vi "sub_angle-limit.vi"(11 "States Out":T1 format="%.4f") -> (3 "Off limit":bool)   [LabVIEW 2018]
uses:
  Model/States.ctl
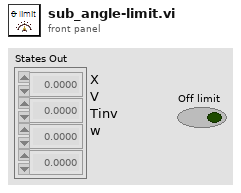
[diagram p1: front panel]
types:
  T1 = typedef "States.ctl" = dbl[]
  T2 = typedef "ctr-ref.ctl" = cluster{"connected":refnum<vi>, "start":refnum<vi>, "read_data":refnum<vi>, "Target":refnum<vi>, "play_type":refnum<vi>, "dt_daq":refnum<vi>, "dt_tcp":refnum<vi>, "timer":refnum<vi>, "States":refnum<vi>, "angle_limit":refnum<vi>, "Initial States":refnum<vi>}
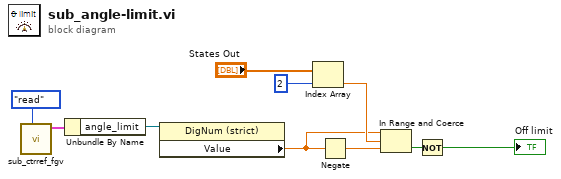
[diagram p0: block diagram]
diagram:
  n1 = call "sub_ctrref_fgv.vi"("cmd"=enum16{"write", "read"}."read") -> ("ctr_out"=w3:T2)  [unwired: 10 in]
  n2 = Unbundle By Name(w3) -> ("angle_limit"=w2:refnum<vi>)
  n3 = property class="DigNum (strict)"(reference=w2) -> ("Value"=w1:dbl)  [unwired: 1 in, 2 out]
  n4 = Index Array(array="States Out", index=2) -> (element=w6:dbl)
  n5 = Negate(x=w1) -> (-x=w8:dbl)
  n6 = In Range and Coerce(upper limit=w1, x=w6, lower limit=w8) -> (In Range?=w9:bool)  [unwired: 1 out]
  n7 = Not(x=w9) -> (.not. x?=→"Off limit":bool)
